vi "Sollwert anpassen T90.vi"(11 "Sollwerteingang":dbl) -> (3 "Sollwertausgang":dbl)   [LabVIEW 2020, in "Allgemein.lvlib"]
uses:
  Allgemein.lvlib
  Aktion FGV T90.ctl
  FGV Komm Status Aktionen.ctl
  Kommunikation mit PC.lvlib
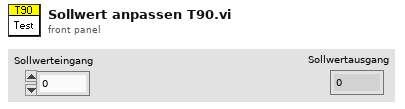
[diagram p1: front panel]
types:
  T1 = typedef "Allgemein.lvlib/Aktion FGV T90.ctl" = enum16{"lesen", "schreiben"}
  T2 = typedef "Kommunikation mit PC.lvlib/FGV Komm Status Aktionen.ctl" = enum16{"lesen", "lebt PC?"}
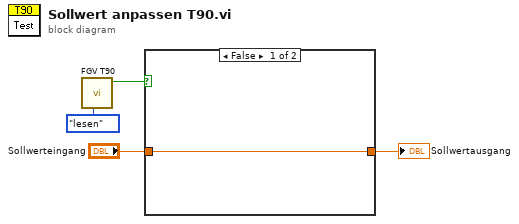
[diagram p0: block diagram]
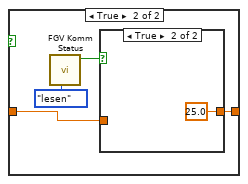
[diagram p2: hidden frame]
diagram:
  n1 = call "FGV T90.vi"("Aktion"=Aktion_FGV_T90."lesen") -> ("T90 aktiv"=w3:bool)  [unwired: 8 in, 2 out]
  n2 = case shown="False" w3 {
    tunnel: "Sollwerteingang" -> [w5 w7]
    tunnel: [w5 w6] -> w1
    frame False {
    }
    frame True {
      n3 = call "FGV Komm Status.vi"("Aktionen"=FGV_Komm_Status_Aktionen."lesen") -> ("lebt PC?"=w8:bool)  [unwired: 10 in]
      n4 = case shown="True" w8 {
        tunnel: w7 -> [w10 _]
        tunnel: [w10 25.0 ("Sollwerteingang")] -> w6
        frame False {
        }
        frame True {
        }
      }
    }
  }
  "Sollwertausgang" <- w1
